vi "AudioStreamer.Trigger.vi"(11 "error in (no error)":errorcluster) -> (15 "error out":errorcluster)   [LabVIEW 2020]
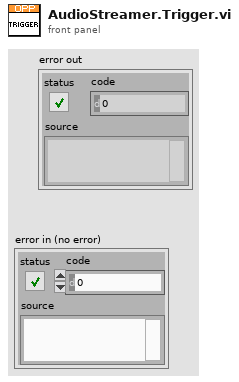
[diagram p1: front panel]
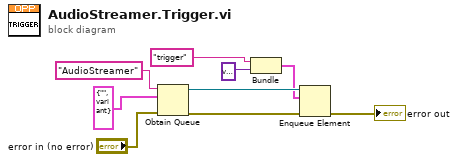
[diagram p0: block diagram]
diagram:
  n1 = Obtain Queue(name (unnamed)="AudioStreamer", element data type=cluster{string, variant} {"", variant}, error in (no error)="error in (no error)") -> (queue out=w6:refnum<queue>, error out=w7:errorcluster)  [unwired: 2 in, 1 out]
  n2 = Bundle("trigger", variant) -> (w3:cluster{string, variant})  [unwired: 1 in]
  n3 = Enqueue Element(queue=w6, element=w3, error in (no error)=w7) -> (error out=→"error out":errorcluster)  [unwired: 1 in, 2 out]
